vi "PressStrainParameters.vi"() -> ()   [LabVIEW 2022 SP3]
panel:
  out "strain %":dbl
  out "depth (mm)":dbl
  out "arc (mm)":dbl
  in  "aperture":dbl
  in  "focal length":dbl
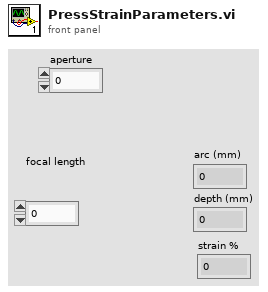
[diagram p1: front panel]
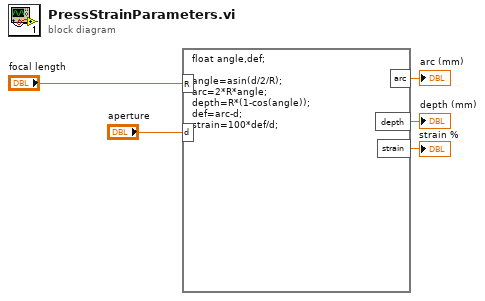
[diagram p0: block diagram]
diagram:
  n1 = formula code="float angle,def;\n\nangle=asin(d/2/R);\narc=2*R*angle;\ndepth=R*(1-cos(angle));\ndef=arc-d;\nstrain=100*def/d;"("R"="focal length", "d"="aperture") -> ("arc"=→"arc (mm)":dbl, "depth"=→"depth (mm)":dbl, "strain"=→"strain %":dbl)
